vi "CommandMotorControl.vi"(11 "Up/Down Control":dbl(slide) min=-1.0 max=1.0 scale=-1.0..1.0) -> ()   [LabVIEW 2017]
uses:
  <vilib>/addons/control/pid/pid.llb/PID (DBL).vi
  <vilib>/addons/control/pid/NI_PID_pid.lvlib
panel:
  out "output":dbl format="%.2f"
  in  "PID gains":T1={"proportional gain (Kc)"=1.0, "integral time (Ti, min)"=0.01, "derivative time (Td, min)"=0.0} {"derivative time (Td, min)" format="%.3f"; "integral time (Ti, min)" format="%.3f"; "proportional gain (Kc)" format="%.3f"}
  in  "Number of Motors":u8(ring) items=["4", "6"]
  out "Array":dbl[](array[numeric])
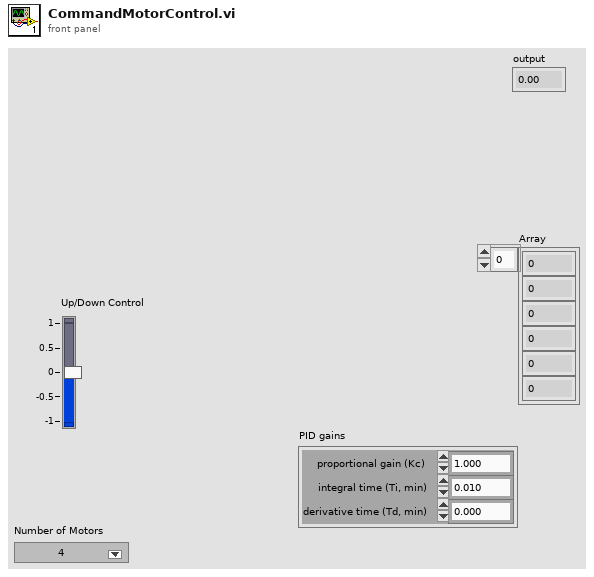
[diagram p1: front panel]
types:
  T1 = cluster{"proportional gain (Kc)":dbl, "integral time (Ti, min)":dbl, "derivative time (Td, min)":dbl}
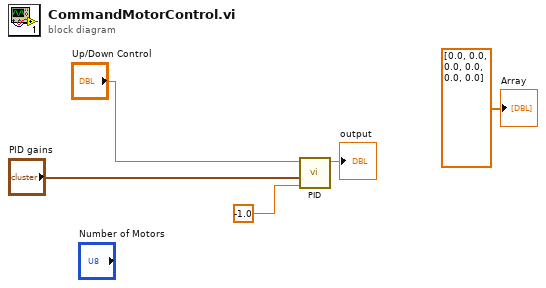
[diagram p0: block diagram]
diagram:
  n1 = call-poly <vilib>:"PID.vi"("dt (s)"=-1.0, "PID gains"="PID gains", "setpoint"="Up/Down Control") -> ("output"=→"output":dbl)  [unwired: 7 in, 1 out]
  "Array" <- dbl[] [0.0, 0.0, 0.0, 0.0, 0.0, 0.0]
